vi "Get Template.vi"(8 "에러 입력":errorcluster caption="에러 입력(에러 없음)", 9 "세부분류코드":string) -> (0 "에러 출력":errorcluster, 3 "Templates Path":path)   [LabVIEW 2020]
uses:
  Controls/Cmd_File path.ctl
  Controls/Cmd_File Type.ctl
  <vilib>/Utility/error.llb/Error Cluster From Error Code.vi
  <vilib>/ErrorRing/Error Ring.xnode
  <vilib>/FTP/NI_FTP.lvlib
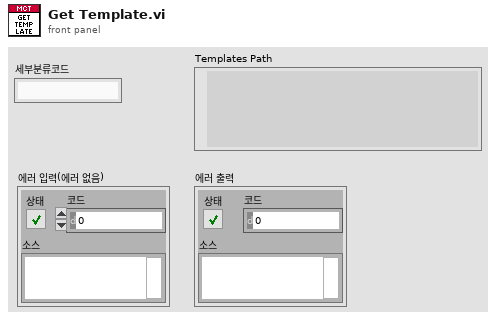
[diagram p1: front panel]
types:
  T1 = typedef "Cmd_File Type.ctl" = enum16{"엑셀", "엑셀(2003)", "텍스트", "설정", "2진", "VI", "CSV", "LOG", "폴더"}
  T2 = typedef "Cmd_File path.ctl" = enum16{"에러로그", "데이터파일경로", "성적서원본", "지난성적서", "Data Files", "경로생성", "Updater", "Template", "설정파일경로", "FTP Upload", "Update 경로", "어플리케이션"}
  T3 = typedef "NI_FTP.lvlib/FTP Session.ctl" = refnum<k5>
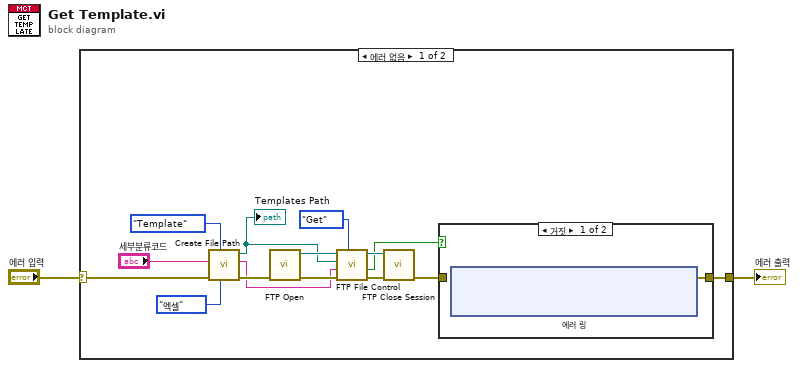
[diagram p0: block diagram]
diagram:
  n1 = case shown="에러 없음" "에러 입력" {
    selector: "에러 입력" -> [w8 w25]
    tunnel: [w17 w25] -> w2
    frame No Error {
      n2 = call "Create File Path.vi"("파일타입"=Cmd_File_Type."엑셀", "항목"=Cmd_File_path."Template", "에러 입력"=w8, "문자열 in"="세부분류코드") -> ("error out"=w7:errorcluster, "문자열 out"=w3:string, "파일경로"=w4:path)  [unwired: 4 in, 1 out]
      "Templates Path" <- w4
      n3 = call "FTP Open.vi"("에러 입력(에러 없음)"=w7) -> ("에러 출력"=w15:errorcluster, "TCP 네트워크 연결 출력"=w16:T3)  [unwired: 9 in]
      n4 = call "FTP File Control.vi"("Comm"=enum16{"Get", "Put"}."Get", "에러 입력"=w15, "원격경로"=w3, "로컬경로"=w4, "TCP 네트워크 연결 입력"=w16) -> ("에러 출력"=w13:errorcluster, "파일존재?"=w11:bool, "TCP 네트워크 연결 출력"=w14:T3)  [unwired: 2 in, 2 out]
      n5 = call <vilib>:"FTP Close Session.vi"("error in (no error)"=w13, "ftp session"=w14) -> ("error out"=w12:errorcluster)  [unwired: 6 in, 3 out]
      n6 = case shown="거짓" w11 {
        tunnel: [w18 w24] -> w17
        tunnel: w12 -> [_ w24]
        frame False {
          n7 = xnode "에러 링"() -> ("에러 출력"=w18:errorcluster)
        }
        frame True {
        }
      }
    }
    frame Error {
    }
  }
  "에러 출력" <- w2
